vi "Label_Prefix.vi"() -> (0 "Label Prefix String":string)   [LabVIEW 2016, in "Hardware.lvlib" / "Motor.lvlib" / "Motor Configuration.lvclass"]
uses:
  <userlib>/Common Components/Hardware/Motor/Motor Config/Motor Configuration.lvclass
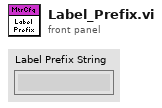
[diagram p1: front panel]
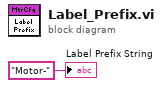
[diagram p0: block diagram]
diagram:
  "Label Prefix String" <- "Motor-" ("Label Prefix String")
